vi "Autonomous Logging.vi"() -> ()   [LabVIEW 2015]
uses:
  <vilib>/Rock Robotics/WPI/DriverStation/WPI_DriverStationRobotMode2.ctl
  Global Variables/Logging Data.vi
  Global Variables/refnum names.vi
  Global Variables/Sensor Data.vi
  Global Variables/Vision Processing Data.vi
  Global Variables/Calibrations.vi
panel:
  out "System Time":string
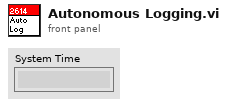
[diagram p1: front panel]
types:
  T1 = typedef "WPI_DriverStationRobotMode2.ctl" = enum16{"Autonomous Disabled", "Autonomous Enabled", "Teleop Disabled", "Teleop Enabled", "Disconnected", "Finish", "Test Disabled", "Test Enabled", "Emergency Stopped"}
  T2 = typedef "Autonomous Command Names.ctl" = enum16{"No Op", "Drive Time", "Run Motion Profile", "Turn to Heading", "Turn To Target", "Cross Defense", "Fire", "Wait", "Reset Gyro", "Grabber Setpoints", "Manual Grabber", "Roller", "Autorange Command", "Reposition", "Drive Distance"}
  T3 = cluster{"Param 1":dbl, "Param 2":dbl, "Autonomous Command Name":T2, "Concurrent":bool, "Param 3":dbl, "Param 4":string}
  T4 = cluster{"Distance (ft)":dbl, "Center":cluster{dbl, dbl}, "Normalized Rect":cluster{"Numeric":dbl, "Numeric 2":dbl, "Numeric 3":dbl, "Numeric 5":dbl}}[]
  T5 = typedef "WPI_MotorControlDeviceRef.ctl" = cluster{"DeviceStatus":errorcluster, "Type":T6, "PWM":cluster{"PWM Channel":T7, "DeadBand":T8}, "CAN":cluster{"Device Number":u8, "Control Mode":T9, "Semaphore":T10, "Max Vout":dbl, "TalonSRX Control Mode":T11}, "Invert":bool}
  T6 = typedef "WPI_MotorControlType.ctl" = enum16{"PWM", "CAN", "CANTalonSRX"}
  T7 = typedef "FPGA_DIOPWMChannel.ctl" = enum8{"PWM 0", "PWM 1", "PWM 2", "PWM 3", "PWM 4", "PWM 5", "PWM 6", "PWM 7", "PWM 8", "PWM 9", "PWM MXP 0", "PWM MXP 1", "PWM MXP 2", "PWM MXP 3", "PWM MXP 4", "PWM MXP 5", "PWM MXP 6", "PWM MXP 7", "PWM MXP 8", "PWM MXP 9", "Invalid"}
  T8 = typedef "WPI_PWMDeadband.ctl" = cluster{"Name":string, "maxPositivePwm":i32, "minPositivePwm":i32, "centerPwm":i32, "maxNegativePwm":i32, "minNegativePwm":i32, "angularRange":u16}
  T9 = typedef "WPI_CANJaguar_ControlMode.ctl" = enum8{"Percent VBus", "Current", "Speed", "Position", "Voltage"}
  T10 = typedef "Semaphore RefNum" = refnum<k1>
  T11 = typedef "WPI_CANTalonSRX_APIControlMode.ctl" = enum8{"Percent VBus", "Speed", "Position", "Slave", "Unchanged / Invalid", "Voltage Compensation", "Current", "Motion Profile"}
  T12 = typedef "WPI_CANTalonSRX_GlobalStatus.ctl" = cluster{"Applied Throttle":dbl, "Module Enabled":bool, "CAN Error":errorcluster, "Closed Loop Error":dbl, "Forward Limit Switch Closed":bool, "Reverse Limit Switch Closed":bool, "Sensor Position":dbl, "Sensor Velocity":dbl, "Current":dbl, "Sticky Fault - Over Temp":bool, "Sticky Fault - Under Voltage":bool, "Sticky Fault - Forward Limit":bool, "Sticky Fault - Reverse Limit":bool, "Sticky Fault - Forward Soft Limit":bool, "Sticky Fault - Reverse Soft Limit":bool, "Brake is Enabled":bool, "Encoder Position":dbl, "Encoder Velocity":dbl, "Encoder Index Count":dbl, "Encoder A Pin State":bool, "Encoder B Pin State":bool, "Encoder Index Pin State":bool, "Analog In":dbl, "Analog In Velocity":dbl, "Temperature (C)":dbl, "Battery Voltage":dbl, "Control 5 Is Supported":bool, "Current Profile Slot Select":dbl, "Pos Div 8":bool, "Vel Div 4":bool, "Pulse Width Position":i32, "Pulse Width Velocity":i32, "Pulse Width Rise To Rise (us)":i32, "Pulse Width Rise To Fall (us)":i32, "Mot Prof Active Is Under Run":bool, "Mot Prof Active Has Under Run":bool, "Mot Prof Active Is Last":bool, "Mot Prof Active Velocity Only":bool, "Mot Prof Active Is Valid":bool, "Mot Prof Buffer Is Full":bool, "Mot Prof Active Profile Slot Select":i32, "Mot Prof NextID":i32, "Mot Prof Count":i32, "Mot Prof Active Velocity":dbl, "Mot Prof Active Position":dbl, "Mot Prof Output Enable":i32}
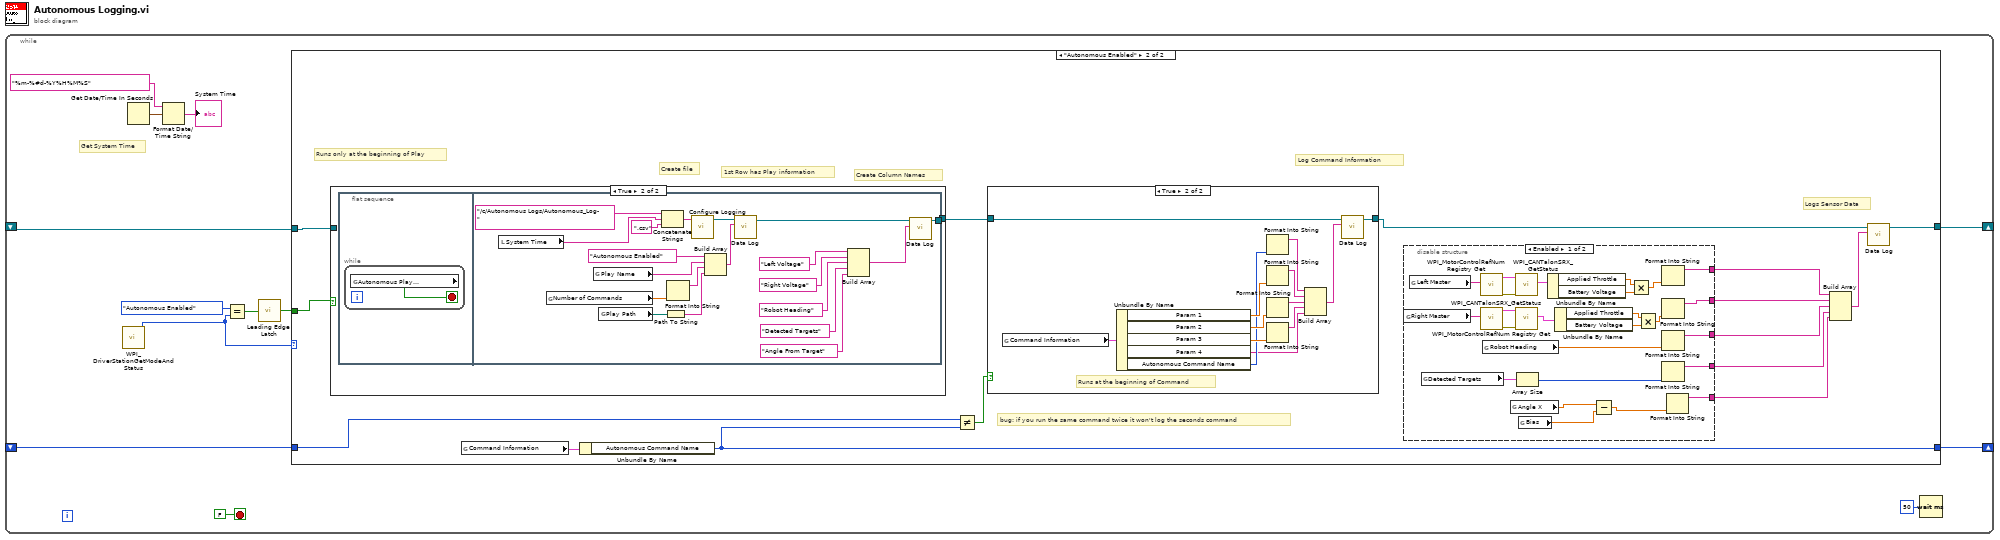
[diagram p0: block diagram]
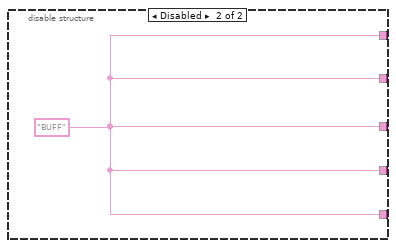
[diagram p5: hidden frame]
diagram:
  n1 = while {
    shift-right: [w11] -> _
    shift-left: _ -> [w10]
    shift-right: [w3] -> _
    shift-left: _ -> [w2]
    stop <- FALSE stop-if-true
    # "Get System Time"
    n2 = call <vilib>:"WPI_DriverStationGetModeAndStatus.vi"() -> ("Robot Mode"=w6:T1)  [unwired: 10 in, 1 out]
    n3 = Get Date/Time In Seconds() -> (seconds since 1Jan1904=w8:timestamp)
    n4 = Format Date/Time String(time format string (%c)="%m-%#d-%Y%H%M%S", seconds (now)=w8) -> (date/time string=→"System Time":string)  [unwired: 1 in]
    n5 = Equal?(x=WPI_DriverStationRobotMode2."Autonomous Enabled" ("Robot Mode"), y=w6) -> (x = y?=w5:bool)
    n6 = call "Leading Edge Latch.vi"("Input"=w5) -> ("Output"=w4:bool)
    n7 = case shown="\"Autonomous Enabled\"" w6 {
      tunnel: [_ w27] -> w11
      tunnel: w10 -> [_ w26]
      tunnel: w4 -> [_ w18]
      tunnel: [_ w19] -> w3
      tunnel: w2 -> [_ w15]
      frame "Autonomous Disabled", Default {
      }
      frame "Autonomous Enabled" {
        # "Runs only at the beginning of Play"
        # "bug: if you run the same command twice it won't log the seconds command"
        # "Create Column Names"
        # "1st Row has Play information"
        # "Log Command Information"
        # "Create file"
        # "Logs Sensor Data"
        n8 = case shown="True" w18 {
          tunnel: [w43 w44] -> w17
          tunnel: w15 -> [w43 _]
          frame False {
          }
          frame True {
            n9 = flat-sequence {
              tunnel: [w48] -> w44
              frame #0 {
                n10 = while {
                  stop <- w45 stop-if-true
                  n11 = global read "Logging Data.vi" "Autonomous Play\nRead"() -> (w45:bool)
                }
              }
              frame #1 {
                n12 = local read "System Time"() -> (w46:string)
                n13 = global read "Logging Data.vi" "Number of Commands"() -> (w61:dbl)
                n14 = global read "Logging Data.vi" "Play Name"() -> (w59:string)
                n15 = global read "Logging Data.vi" "Play Path"() -> (w58:path)
                n16 = Concatenate Strings("/c/Autonomous Logs/Autonomous_Log- " ("time format string (%c)"), w46, ".csv" ("string")) -> (w64:string)
                n17 = Path To String(path=w58) -> (string=w57:string)
                n18 = Format Into String(w61) -> (resulting string=w60:string)  [unwired: 3 in, 1 out]
                n19 = call "Configure Logging.vi"("File Path/File Name"=w64) -> ("refnum out"=w63:refnum<file>)  [unwired: 10 in]
                n20 = Build Array("Autonomous Enabled", w59, w60, w57) -> (w56:string[])
                n21 = call "Data Log.vi"("Data In"=w56, "File Reference In"=w63) -> ("File Reference Out"=w49:refnum<file>)  [unwired: 9 in]
                n22 = Build Array("Left Voltage", "Right Voltage", "Robot Heading", "Detected Targets", "Angle From Target") -> (w50:string[])
                n23 = call "Data Log.vi"("Data In"=w50, "File Reference In"=w49) -> ("File Reference Out"=w48:refnum<file>)  [unwired: 9 in]
              }
            }
          }
        }
        n24 = global read "Logging Data.vi" "Command Information"() -> (w28:T3)
        n25 = Unbundle By Name(w28) -> ("Autonomous Command Name"=w27:T2)
        n26 = Not Equal?(x=w26, y=w27) -> (x != y?=w14:bool)
        n27 = case shown="True" w14 {
          tunnel: w17 -> [w29 w31]
          tunnel: [w29 w30] -> w16
          frame False {
            # "Check File reference\ndefault value.\n\nIf not use shift register to pass back"
          }
          frame True {
            # "Runs at the beginning of Command"
            n28 = global read "Logging Data.vi" "Command Information"() -> (w37:T3)
            n29 = Unbundle By Name(w37) -> ("Param 1"=w42:dbl, "Param 2"=w41:dbl, "Param 3"=w40:dbl, "Param 4"=w36:string, "Autonomous Command Name"=w39:T2)
            n30 = Format Into String(w39) -> (resulting string=w32:string)  [unwired: 3 in, 1 out]
            n31 = Format Into String(w42) -> (resulting string=w33:string)  [unwired: 3 in, 1 out]
            n32 = Format Into String(w41) -> (resulting string=w34:string)  [unwired: 3 in, 1 out]
            n33 = Format Into String(w40) -> (resulting string=w35:string)  [unwired: 3 in, 1 out]
            n34 = Build Array(w32, w33, w34, w35, w36) -> (w38:string[])
            n35 = call "Data Log.vi"("Data In"=w38, "File Reference In"=w31) -> ("File Reference Out"=w30:refnum<file>)  [unwired: 9 in]
          }
        }
        n36 = disable-structure shown="Enabled" {
          disable-tunnel: [w84 w91] -> w25
          disable-tunnel: [w83 w91] -> w24
          disable-tunnel: [w81 w91] -> w23
          disable-tunnel: [w78 w91] -> w22
          disable-tunnel: [w77 w91] -> w20
          frame Enabled {
            n37 = global read "refnum names.vi" "Right Master"() -> (w88:string)
            n38 = global read "refnum names.vi" "Left Master"() -> (w89:string)
            n39 = global read "Vision Processing Data.vi" "Detected Targets"() -> (w80:T4)
            n40 = call <vilib>:"WPI_MotorControlRefNum Registry Get.vi"("refnum name"=w89) -> ("error out"=w85:errorcluster, "MotorControlDevRef"=w90:T5)  [unwired: 9 in]
            n41 = call <vilib>:"WPI_MotorControlRefNum Registry Get.vi"("refnum name"=w88) -> ("error out"=w86:errorcluster, "MotorControlDevRef"=w87:T5)  [unwired: 9 in]
            n42 = global read "Sensor Data.vi" "Robot Heading"() -> (w82:dbl)
            n43 = global read "Vision Processing Data.vi" "Angle X"() -> (w68:dbl)
            n44 = call <vilib>:"WPI_CANTalonSRX_GetStatus.vi"("error in (no error)"=w85, "CAN Talon SRX Ref"=w90) -> ("Talon SRX Status"=w76:T12)  [unwired: 7 in, 2 out]
            n45 = call <vilib>:"WPI_CANTalonSRX_GetStatus.vi"("error in (no error)"=w86, "CAN Talon SRX Ref"=w87) -> ("Talon SRX Status"=w70:T12)  [unwired: 7 in, 2 out]
            n46 = Array Size(array=w80) -> (size(s)=w79:i32)
            n47 = global read "Calibrations.vi" "Bias"() -> (w67:dbl)
            n48 = Unbundle By Name(w76) -> ("Applied Throttle"=w74:dbl, "Battery Voltage"=w73:dbl)
            n49 = Unbundle By Name(w70) -> ("Applied Throttle"=w72:dbl, "Battery Voltage"=w71:dbl)
            n50 = Subtract(x=w68, y=w67) -> (x-y=w66:dbl)
            n51 = Multiply(x=w74, y=w73) -> (x*y=w75:dbl)
            n52 = Multiply(x=w72, y=w71) -> (x*y=w69:dbl)
            n53 = Format Into String(w75) -> (resulting string=w84:string)  [unwired: 3 in, 1 out]
            n54 = Format Into String(w69) -> (resulting string=w83:string)  [unwired: 3 in, 1 out]
            n55 = Format Into String(w82) -> (resulting string=w81:string)  [unwired: 3 in, 1 out]
            n56 = Format Into String(w79) -> (resulting string=w78:string)  [unwired: 3 in, 1 out]
            n57 = Format Into String(w66) -> (resulting string=w77:string)  [unwired: 3 in, 1 out]
          }
          frame Disabled {
            w91 = "BUFF" ("string")
          }
        }
        n58 = Build Array(w25, w24, w23, w22, w20) -> (w21:string[])
        n59 = call "Data Log.vi"("Data In"=w21, "File Reference In"=w16) -> ("File Reference Out"=w19:refnum<file>)  [unwired: 9 in]
      }
    }
    n60 = Wait (ms)(milliseconds to wait=u32 50) -> ()  [unwired: 1 out]
  }
